vi "Untitled 1.vi"() -> ()   [LabVIEW 2016]
panel:
  out "Array 3":u32[](array[colorbox])
  in  "Array 2":u16[](array[numeric])
  out "timing":u32
  in  "String":string
  out "Luminance":u8
  out "Hue":u8
  out "Array":u16[](array[numeric])
  out "x-1":u16
  in  "Numeric":u16
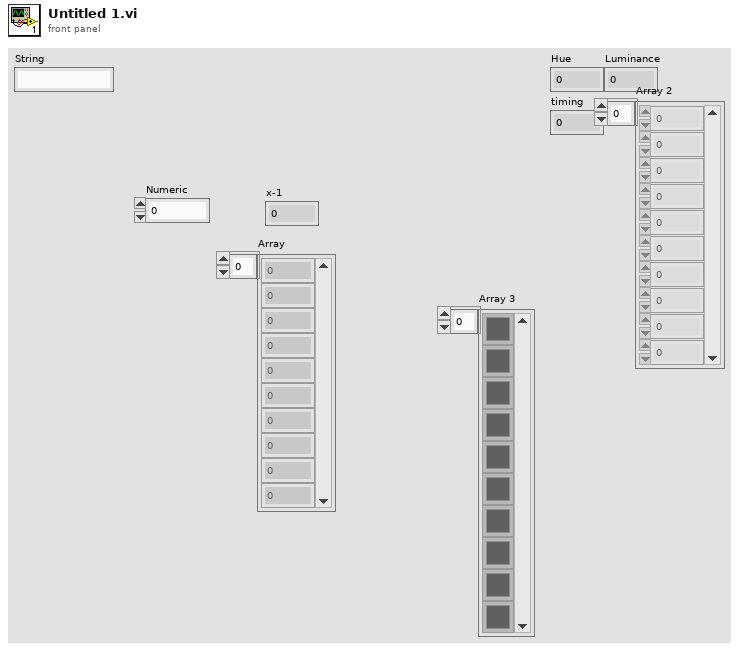
[diagram p1: front panel]
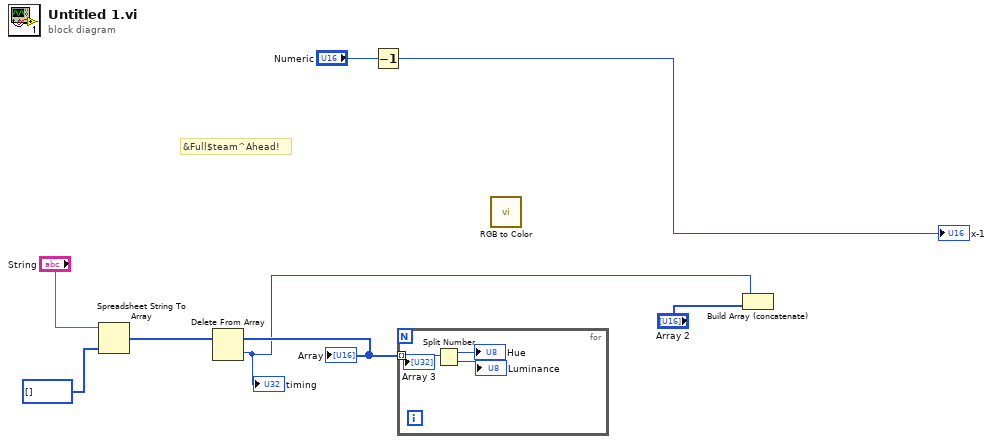
[diagram p0: block diagram]
diagram:
  # "&Full$team^Ahead!"
  n1 = Spreadsheet String To Array(format string="String", array type (2D Dbl)=u32[] []) -> (array=w4:u32[])  [unwired: 2 in]
  n2 = Delete From Array(array=w4) -> (deleted portion=w2:u32, array with subset deleted=w3:u32[])  [unwired: 2 in]
  "Array" <- w3
  "timing" <- w2
  n3 = Decrement(x="Numeric") -> (x-1=→"x-1":u16)
  n4 = for {
    tunnel: w3 -> [w11] mode=indexing
    n5 = Split Number(x=w11) -> (hi(x)=→"Hue":u16, lo(x)=→"Luminance":u16)
  }
  n6 = call <vilib>:"RGB to Color.vi"() -> ()  [unwired: 3 in, 1 out]
  n7 = Build Array (concatenate)(w2, "Array 2") -> ()  [unwired: 1 out]
